vi "SetLeds.vi"() -> (0 "Array":T1[](array[typedef]) {"Led_offH" format="%x"; "Led_offL" format="%x"; "Led_onH" format="%x"; "Led_onL" format="%x"})   [LabVIEW 2022 SP3, in "PCA9685.lvlib" / "PCA.lvclass"]
uses:
  PCA.lvclass
  PCA.lvclass/PCA.ctl
  typedefs/Led.ctl
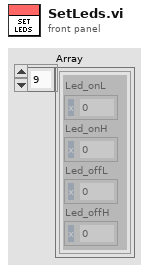
[diagram p1: front panel]
types:
  T1 = typedef "PCA9685.lvlib/PCA.lvclass/Led.ctl" = cluster{"Led_onL":i8, "Led_onH":i8, "Led_offL":i8, "Led_offH":i8}
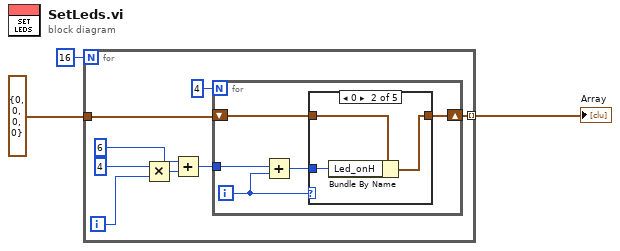
[diagram p0: block diagram]
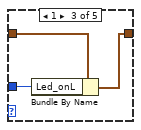
[diagram p3: hidden frame]
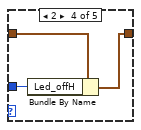
[diagram p4: hidden frame]
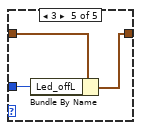
[diagram p5: hidden frame]
diagram:
  n1 = for {
    N: 16 -> [_]
    tunnel: T1 {"Led_onL"=0, "Led_onH"=0, "Led_offL"=0, "Led_offH"=0} ("LED") -> [w11]
    tunnel: [w10] -> w1 mode=indexing
    i -> [w8]
    n2 = Multiply(x=4, y=w8) -> (x*y=w6:i32)
    n3 = Add(x=6, y=w6) -> (x+y=w5:i32)
    n4 = for {
      N: 4 -> [_]
      tunnel: w5 -> [w13]
      shift-right: [w15] -> w10
      shift-left: w11 -> [w16]
      i -> [w14]
      n5 = Add(x=w13, y=w14) -> (x+y=w12:i32)
      n6 = case shown="0" w14 {
        tunnel: w16 -> [w17 w20 w23 w26 w29]
        tunnel: [w17 w18 w21 w24 w28] -> w15
        tunnel: w12 -> [_ w19 w22 w25 w27]
        frame Default {
        }
        frame 0 {
          n7 = Bundle By Name(cluster=w20, "Led_onH"=w19) -> (w18:T1)
        }
        frame 1 {
          n8 = Bundle By Name(cluster=w23, "Led_onL"=w22) -> (w21:T1)
        }
        frame 2 {
          n9 = Bundle By Name(cluster=w26, "Led_offH"=w25) -> (w24:T1)
        }
        frame 3 {
          n10 = Bundle By Name(cluster=w29, "Led_offL"=w27) -> (w28:T1)
        }
      }
    }
  }
  "Array" <- w1
